vi "LV2015_PC_DEMO Build SD Card File.vi"() -> ()   [LabVIEW 2016]
uses:
  TypeDefs/Cluster_Page Data.ctl
panel:
  out "SD Card File Array":T1[](array[typedef])
  in  "File Name":string="MotionDemo"
  in  "Test file Folder":path
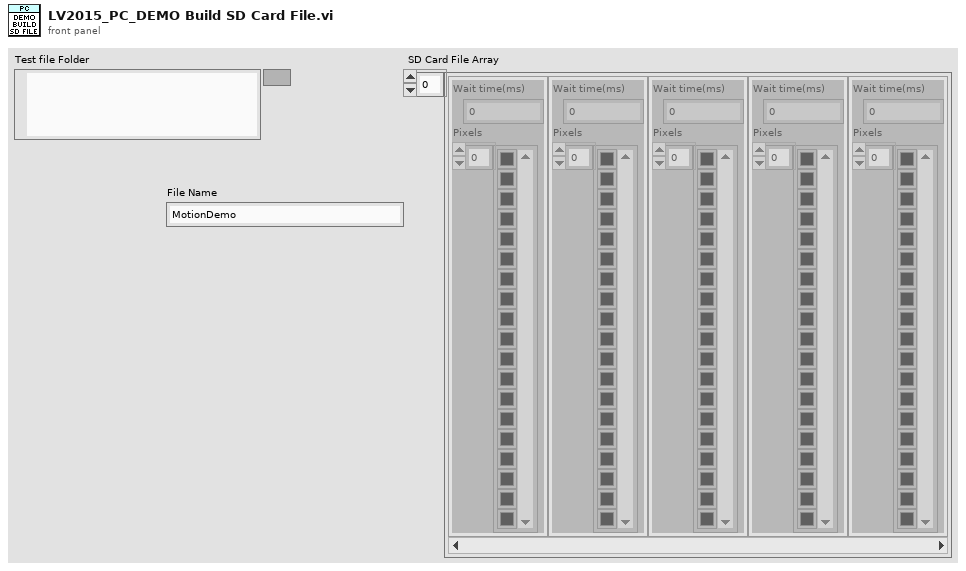
[diagram p1: front panel]
types:
  T1 = typedef "Cluster_Page Data.ctl" = cluster{"Wait time(ms)":u32, "Pixels":u32[]}
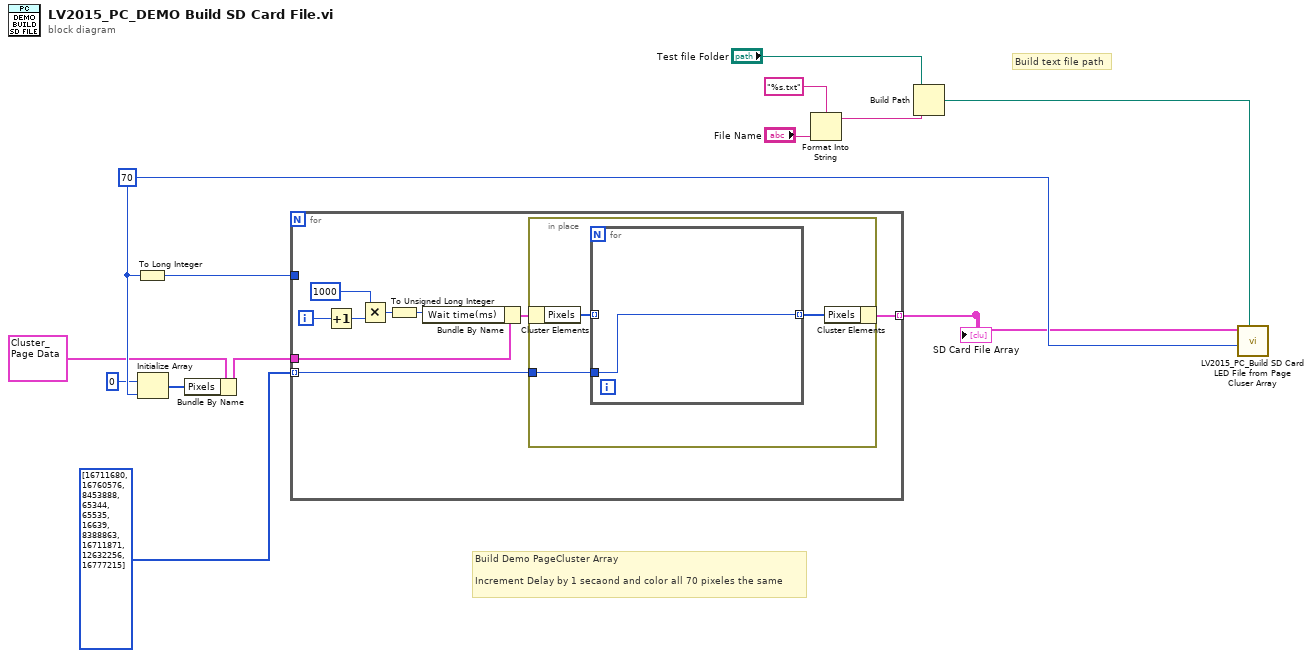
[diagram p0: block diagram]
diagram:
  w12 = u32 70 ("pixel Count")
  # "Build text file path"
  # "Build Demo PageCluster Array\n\nIncrement Delay by 1 secaond and color all 70 pixeles the same"
  n1 = To Long Integer(number=w12) -> (32bit integer=w13:i32)
  n2 = Initialize Array(u32 0 ("pixel Count"), w12) -> (w8:u32[])
  n3 = Bundle By Name(cluster=T1 {"Wait time(ms)"=0, "Pixels"=[0, 0, 0, 0, 0, 0, 0, 0, 0, 0, 0, 0, 0, 0, 0, 0, 0, 0, 0, 0, 0, 0, 0, 0, 0, 0, 0, 0, 0, 0, 0, 0, 0, 0, 0, 0, 0, 0, 0, 0, 0, 0, 0, 0, 0, 0, 0, 0, 0, 0, 0, 0, 0, 0, 0, 0, 0, 0, 0, 0, 0, 0, 0, 0, 0, 0, 0, 0, 0, 0]} ("Page Data"), "Pixels"=w8) -> (w9:T1)
  n4 = for {
    tunnel: w13 -> [_]
    tunnel: w9 -> [w22]
    tunnel: [w15] -> w7 mode=indexing
    tunnel: u32[] [16711680, 16760576, 8453888, 65344, 65535, 16639, 8388863, 16711871, 12632256, 16777215] ("Pixels") -> [w14] mode=indexing
    i -> [w21]
    n5 = Increment(x=w21) -> (x+1=w20:i32)
    n6 = Multiply(x=1000, y=w20) -> (x*y=w18:i32)
    n7 = To Unsigned Long Integer(number=w18) -> (unsigned 32bit integer=w17:u32)
    n8 = Bundle By Name(cluster=w22, "Wait time(ms)"=w17) -> (w16:T1)
    n9 = in-place {
      in-place-border: w14 -> [w23]
      n10 = in-place-cluster #1(w16) -> ("Pixels"=w25:u32[])
      n11 = for {
        tunnel: w25 -> [_] mode=indexing
        tunnel: [w26] -> w24 mode=indexing
        tunnel: w23 -> [w26]
      }
      n12 = in-place-cluster #1("Pixels"=w24) -> (w15:T1)
    }
  }
  "SD Card File Array" <- w7
  n13 = Format Into String(format string="%s.txt", "File Name") -> (resulting string=w4:string)  [unwired: 2 in, 1 out]
  n14 = Build Path(base path="Test file Folder", name or relative path=w4) -> (appended path=w2:path)
  n15 = call "LV2015_PC_Build SD Card LED File from Page Cluser Array.vi"("file path (dialog if empty)"=w2, "pixel Count"=w12, "LED File Array"=w7) -> ()  [unwired: 9 in]
